vi "eTdsBLE_Test.vi"() -> ()   [LabVIEW 2013]
uses:
  D:/GitHub/GT-Bionics/TDS-HM/Labview Code/C# BLE Interface/eTDS BLE Interface/TdsBleInterface for LV/TdsForLV/TdsForLV/bin/TdsForLV.dll
  TdsForLV/TdsForLV/bin/TdsForLV.dll
panel:
  in  "stop":bool
  out "BleDataArray":u8[](array[numeric])
  out "error out":errorcluster
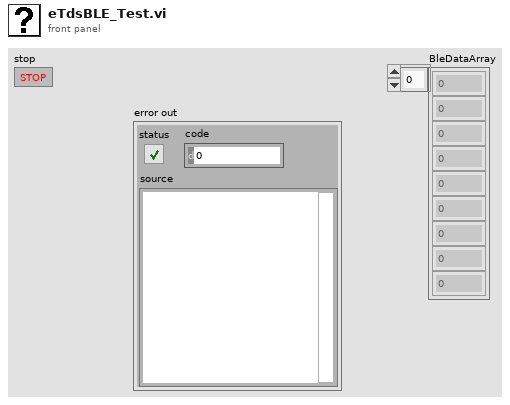
[diagram p1: front panel]
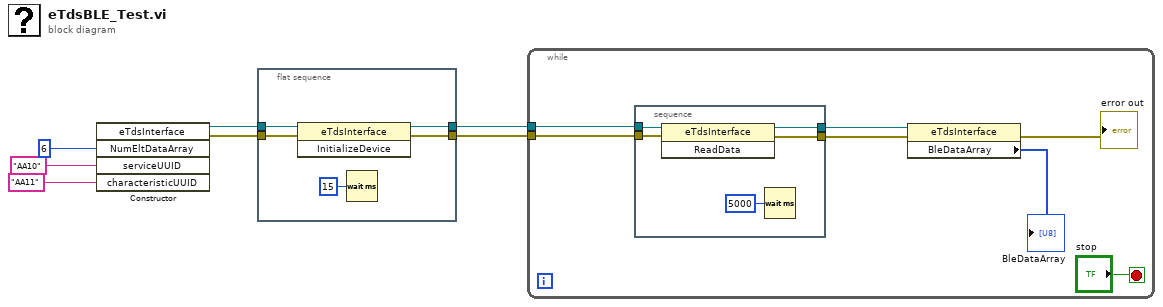
[diagram p0: block diagram]
diagram:
  n1 = constructor class="eTdsInterface"("NumEltDataArray"=6, "serviceUUID"="AA10", "characteristicUUID"="AA11") -> (reference out=w7:refnum<k24>, error out=w6:errorcluster)  [unwired: 3 in, 4 out]
  n2 = flat-sequence {
    tunnel: w7 -> [w12]
    tunnel: w6 -> [w11]
    tunnel: [w10] -> w2
    tunnel: [w9] -> w1
    frame #0 {
      n3 = invoke class="eTdsInterface" method="InitializeDevice"(reference=w12, error in=w11) -> (reference out=w10:refnum<k24>, error out=w9:errorcluster)  [unwired: 1 in, 1 out]
      n4 = Wait (ms)(milliseconds to wait=u32 15) -> ()  [unwired: 1 out]
    }
  }
  n5 = while {
    tunnel: w2 -> [w19]
    tunnel: w1 -> [w13]
    stop <- "stop" stop-if-true
    n6 = stacked-sequence {
      tunnel: w19 -> [w24]
      tunnel: w13 -> [w23]
      tunnel: [w22] -> w16
      tunnel: [w21] -> w15
      frame #0 {
        n7 = invoke class="eTdsInterface" method="ReadData"(reference=w24, error in=w23) -> (reference out=w22:refnum<k24>, error out=w21:errorcluster)  [unwired: 1 in, 1 out]
        n8 = Wait (ms)(milliseconds to wait=u32 5000) -> ()  [unwired: 1 out]
      }
    }
    n9 = property class="eTdsInterface"(reference=w16, error in=w15) -> (error out=→"error out":errorcluster, "BleDataArray"=→"BleDataArray":u8[])  [unwired: 1 out]
  }
